vi "waveInGetNumDevs.vi"(8 "error in (no error)":errorcluster) -> (0 "error out":errorcluster, 3 "numberOfDevices":u32)   [LabVIEW 2011]
uses:
  Windows/System32/winmm.dll
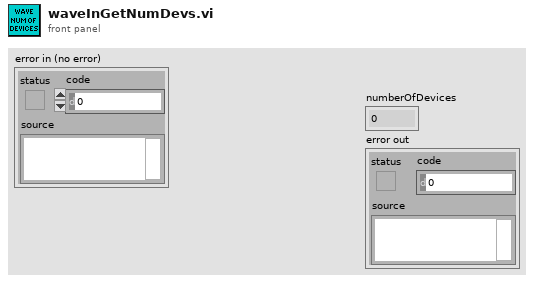
[diagram p1: front panel]
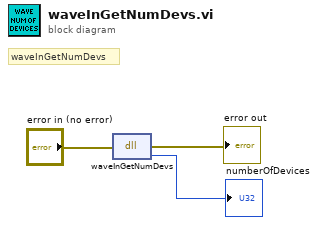
[diagram p0: block diagram]
diagram:
  # "waveInGetNumDevs"
  n1 = dll-call lib="C:/Windows/System32/winmm.dll" fn="waveInGetNumDevs"(error in="error in (no error)") -> (error out=→"error out":errorcluster, "return type"=→"numberOfDevices":u32)  [unwired: 2 in, 1 out]
